vi "Table Select Section Paste From 1D Array.vi"(9 "Paste Value":string[](array[string]), 11 "Table Ref In":refnum<vi>) -> (3 "Table Ref Out":refnum<vi>)   [LabVIEW 2024]
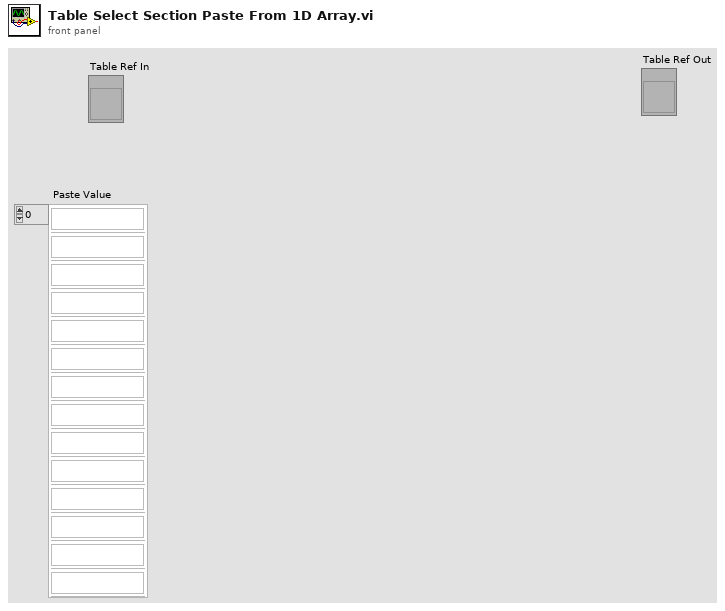
[diagram p1: front panel]
types:
  T1 = typedef "LVRowAndColumnTypeDef.ctl" = cluster{"Row":i32, "Column":i32}
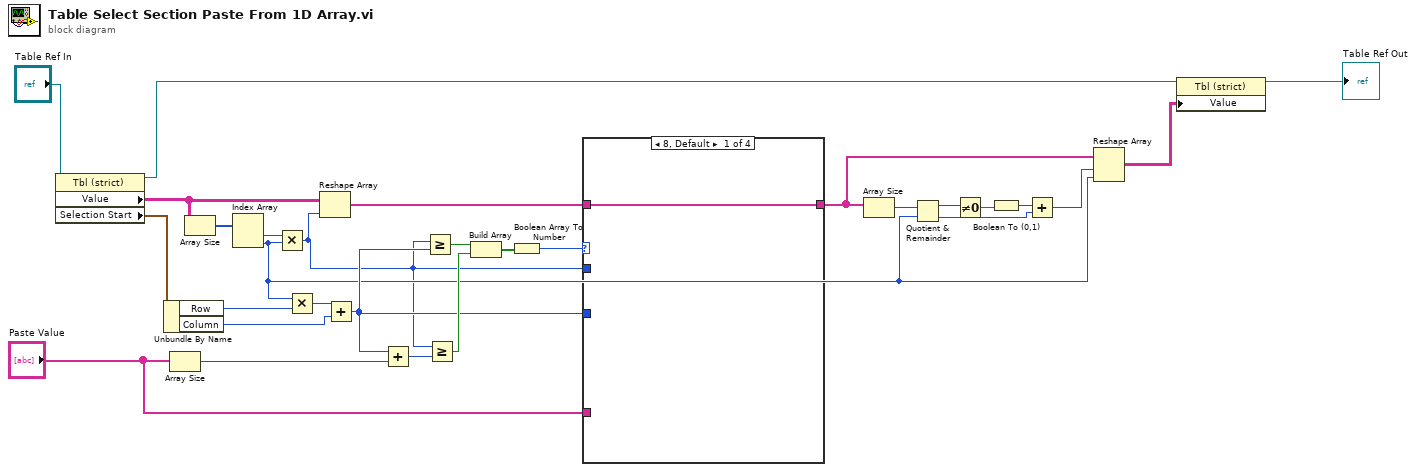
[diagram p0: block diagram]
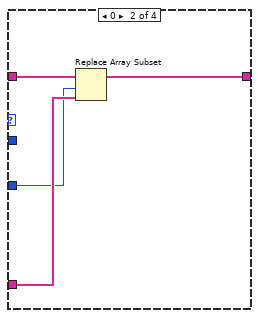
[diagram p2: hidden frame]
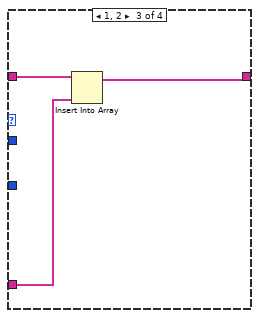
[diagram p3: hidden frame]
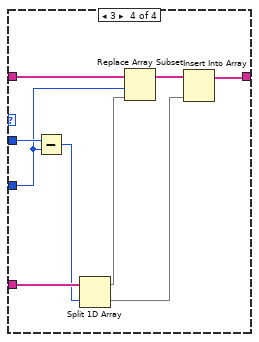
[diagram p4: hidden frame]
diagram:
  n1 = property class="Tbl (strict)"(reference="Table Ref In") -> (reference out=w26:refnum<vi>, "Value"=w25:string[][], "Selection Start"=w29:T1)  [unwired: 1 in, 1 out]
  n2 = Unbundle By Name(w29) -> ("Row"=w23:i32, "Column"=w21:i32)
  n3 = Array Size(array="Paste Value") -> (size(s)=w18:i32)
  n4 = Array Size(array=w25) -> (size(s)=w24:i32[])
  n5 = Index Array(array=w24) -> (element #1=w20:i32, element #2=w3:i32)  [unwired: 2 in]
  n6 = Multiply(x=w20, y=w3) -> (x*y=w1:i32)
  n7 = Multiply(x=w3, y=w23) -> (x*y=w22:i32)
  n8 = Reshape Array(w25, w1) -> (w19:string[])
  n9 = Add(x=w22, y=w21) -> (x+y=w11:i32)
  n10 = Add(x=w11, y=w18) -> (x+y=w16:i32)
  n11 = Greater Or Equal?(x=w1, y=w11) -> (x >= y?=w17:bool)
  n12 = Greater Or Equal?(x=w1, y=w16) -> (x >= y?=w15:bool)
  n13 = Build Array(w17, w15) -> (w14:bool[])
  n14 = Boolean Array To Number(Boolean array=w14) -> (number=w13:u32)
  n15 = case shown="8, Default" w13 {
    tunnel: w19 -> [w30 w34 w37 w43]
    tunnel: "Paste Value" -> [_ w33 w35 w46]
    tunnel: w11 -> [_ w32 _ w42]
    tunnel: [w30 w31 w36 w39] -> w5
    tunnel: w1 -> [_ _ _ w45]
    frame 8, Default {
    }
    frame 0 {
      # "Directly Replace"
      n16 = Replace Array Subset(array=w34, new element=w33, index=w32) -> (w31:string[])
    }
    frame 1, 2 {
      n17 = Insert Into Array(array=w37, new element=w35) -> (w36:string[])  [unwired: 1 in]
    }
    frame 3 {
      n18 = Subtract(x=w45, y=w42) -> (x-y=w44:i32)
      n19 = Split 1D Array(array=w46, index=w44) -> (first subarray=w41:string[], second subarray=w38:string[])
      n20 = Replace Array Subset(array=w43, new element=w41, index=w42) -> (w40:string[])
      n21 = Insert Into Array(array=w40, new element=w38) -> (w39:string[])  [unwired: 1 in]
    }
  }
  n22 = Array Size(array=w5) -> (size(s)=w10:i32)
  n23 = Quotient & Remainder(x=w10, y=w3) -> (x-y*floor(x/y)=w9:i32, floor(x/y)=w6:i32)
  n24 = Not Equal To 0?(x=w9) -> (x != 0?=w8:bool)
  n25 = Boolean To (0,1)(Boolean=w8) -> (0, 1=w7:i16)
  n26 = Add(x=w7, y=w6) -> (x+y=w4:i32)
  n27 = Reshape Array(w5, w4, w3) -> (w2:string[][])
  n28 = property class="Tbl (strict)"(reference=w26, "Value"=w2) -> (reference out=→"Table Ref Out":refnum<vi>)  [unwired: 1 in, 1 out]
